vi "1_3oct_extrator_csv_to_csv.vi"() -> ()   [LabVIEW 2017]
doc: "Permite obtener un archivo CSV de etiquetado automático de secciones de señal. \nIngresa: un archivo CSV que contiene el sample inicial, final y la etiqueta correspondiente.\nUn archivo TDMS que contenga la información del registro de la señal.\nSe debe colocar la dirección del archivo de salida.\nEstablecer el número de samples que contendrá cada parte en que se dividirá la sección.\nAl momento el VI no contempla traslapamiento."
uses:
  <vilib>/Waveform/WDTOps.llb/WDT Get Waveform Subset DBL.vi
  <vilib>/addons/Sound and Vibration/svt_Octave_2014 standard/SVT Third-octave Analysis (1 Ch).vi
  <vilib>/addons/Sound and Vibration/svt_Level/SVT Sound Level (1 Ch).vi
  <vilib>/Utility/file.llb/Write Delimited Spreadsheet (string).vi
  <vilib>/addons/Sound and Vibration/svt_Octave/SoundVib_Octave_2014 standard.lvlib
  <vilib>/addons/Sound and Vibration/svt_Level/SoundVib_SoundLevel.lvlib
panel:
  out "F-format string":string[][](array[string])
  out "Array":dbl[][](array[numeric])
  out "Dynamic Data Type":dbl
  in  "Canal":string[](array[string])=["Sound Pressure_0"]
  out "Para el CSV, excepto fecha y hora":string[][](array[string])
  out "TIEMPOS":timestamp[](array[timestamp])
  out "Objetos por sección.":i32[][](array[numeric])
  out "Objetos":i32[](array[numeric])
  out "Secciones":i32[](array[numeric])
  out "Objetos totales":i32
  in  "frequency range":T1={"low band"=enum."20 Hz", "high band"=enum."20000 Hz"}
  out "TO CSV.":string[][](array[string])
  out "ETIQUETAS":string[](array[string])
  out "BANDAS":dbl[][](array[numeric])
  in  "ETIQUETADO":path=path "C:/Users/CRamos/Documents/MATLAB/etiquetador/csv_OUT/DATOS_caracte.csv"
  out "Objeto actual":i32
  out "Sección Actual":i32
  out "Samples \npor Objeto":waveform(dbl)
  in  "Largo de ventada temporal en N samples":dbl=4410.0
  out "Secciones":waveform(dbl)[](array[waveform])
  out "Multiplot \noctave graph":T2(graph)
  in  "ARCHIVO\nTDMS":path=path "C:/Users/CRamos/Documents/MATLAB/TDMS_files/two_sounds.tdms"
  in  "Archivo de\nreferencias (.csv)":path=path "C:/Users/CRamos/Documents/MATLAB/etiquetador/csv_IN/DATOS.csv"
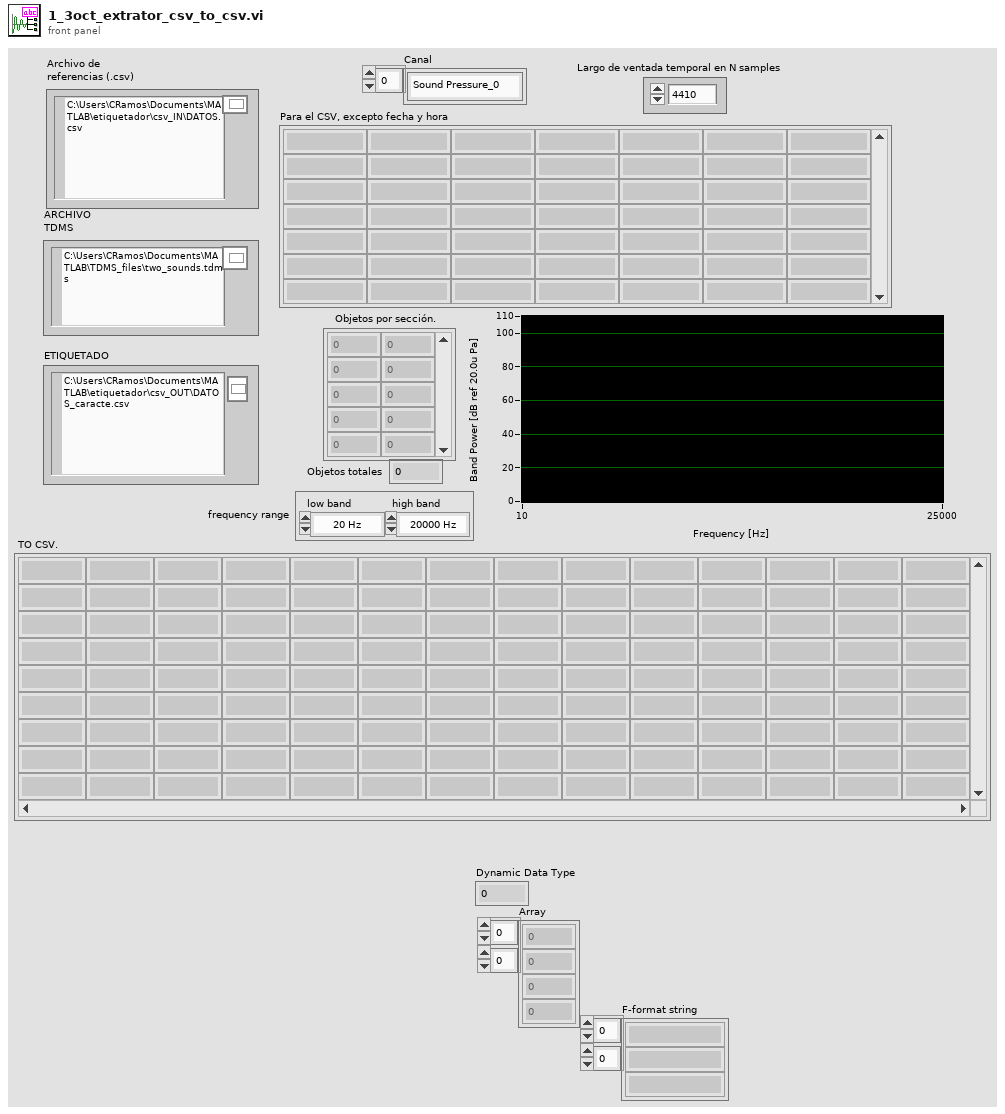
[diagram p1: front panel]
types:
  T1 = cluster{"low band":enum16{"20 Hz", "25 Hz", "31.5 Hz", "40 Hz", "50 Hz", "63 Hz", "80 Hz", "100 Hz", "125 Hz", "160 Hz", "200 Hz", "250 Hz", "315 Hz", "400 Hz", "500 Hz", "630 Hz", "800 Hz", "1000 Hz", "1250 Hz", "1600 Hz", "2000 Hz", "2500 Hz", "3150 Hz", "4000 Hz", "5000 Hz", "6300 Hz", "8000 Hz", "10000 Hz", "12500 Hz", "16000 Hz", "20000 Hz"}, "high band":enum16{"20 Hz", "25 Hz", "31.5 Hz", "40 Hz", "50 Hz", "63 Hz", "80 Hz", "100 Hz", "125 Hz", "160 Hz", "200 Hz", "250 Hz", "315 Hz", "400 Hz", "500 Hz", "630 Hz", "800 Hz", "1000 Hz", "1250 Hz", "1600 Hz", "2000 Hz", "2500 Hz", "3150 Hz", "4000 Hz", "5000 Hz", "6300 Hz", "8000 Hz", "10000 Hz", "12500 Hz", "16000 Hz", "20000 Hz"}}
  T2 = cluster{"nominal frequencies [Hz]":dbl[], "band power":dbl[]}
  T3 = enum16{"open", "open or create", "create or replace", "create", "open (read-only)"}
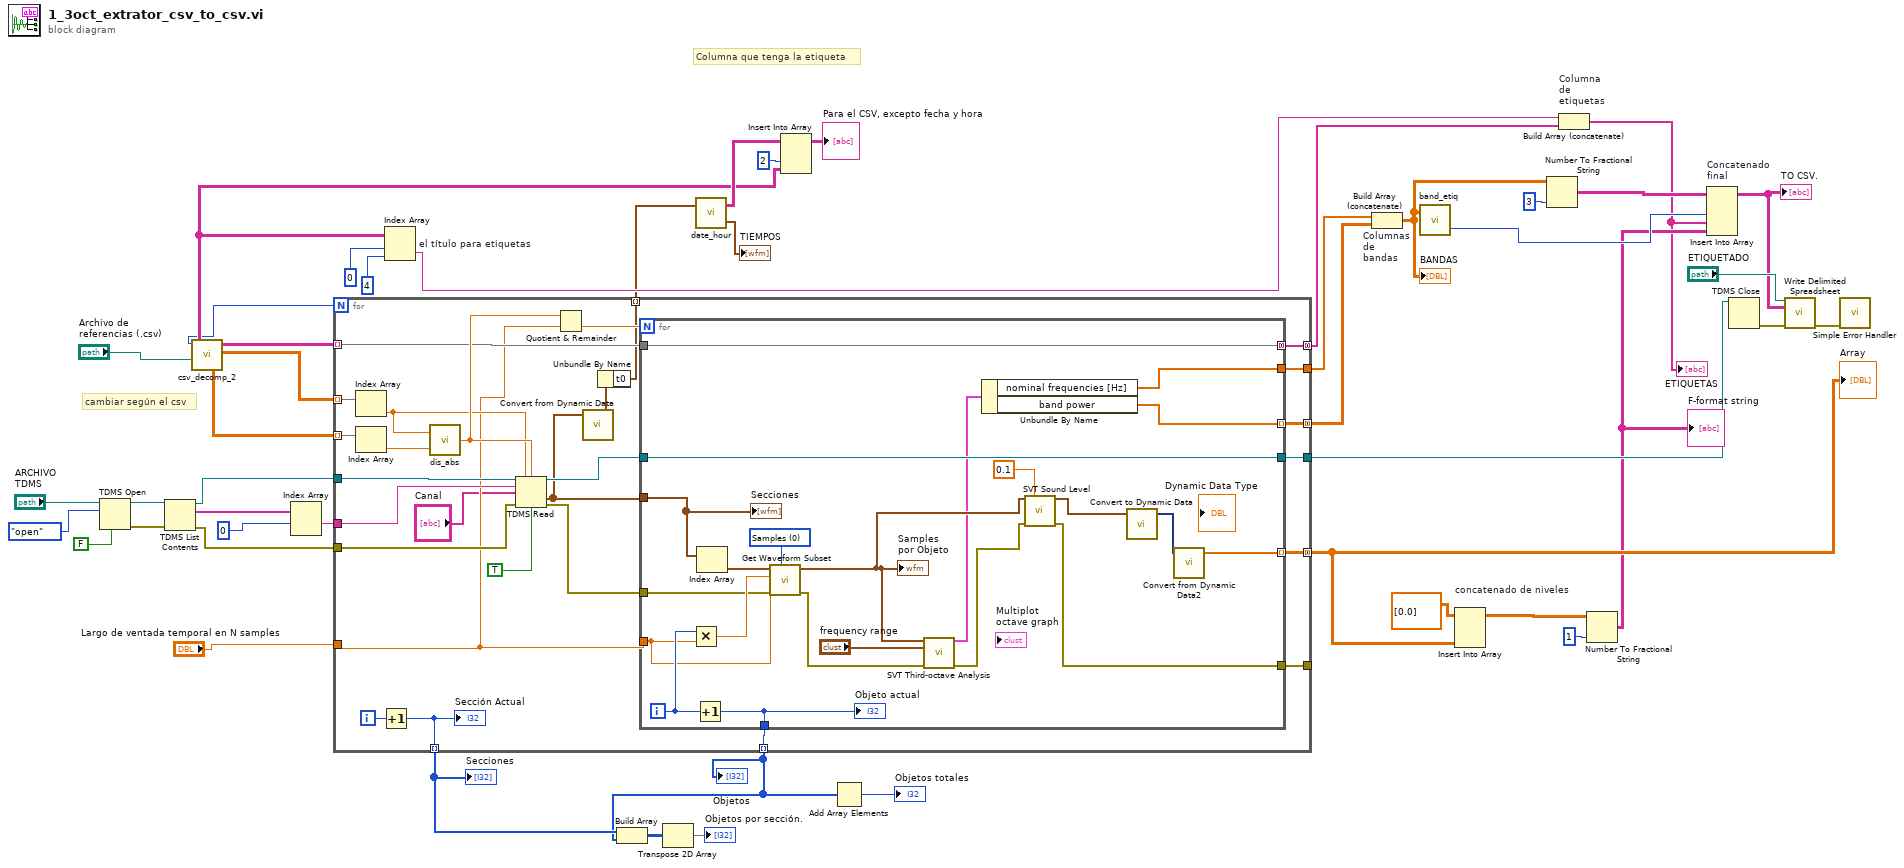
[diagram p0: block diagram]
diagram:
  # "cambiar según el csv"
  # "Columna que tenga la etiqueta"
  n1 = TDMS Open(6:FALSE ("disable buffering? (T)"), 10:T3."open" ("operation (0:open)"), 11:"ARCHIVO\nTDMS") -> (0:w45:errorcluster, 3:w16:refnum<k34>)  [unwired: 4 in]
  n2 = TDMS List Contents(4:w45, 7:w16) -> (0:w14:errorcluster, 2:w15:string[], 3:w44:refnum<k34>)  [unwired: 1 in, 1 out]
  n3 = call "csv_decomp_2.vi"("Archivo de referencias (.csv)"="Archivo de\nreferencias (.csv)") -> ("finales"=w9:dbl[][], "iniciales"=w8:dbl[][], "etiquetas"=w10:string[][], "# dimención"=w11:i32, "Lectura CSV"=w13:string[][])  [unwired: 2 in]
  n4 = Index Array(array=w15, index #1=0 ("index")) -> (element #1=w42:string)  [unwired: 1 in, 1 out]
  n5 = for {
    N: w11 -> [_]
    tunnel: w8 -> [w72] mode=indexing
    tunnel: w9 -> [w73] mode=indexing
    tunnel: w10 -> [w60] mode=indexing
    tunnel: w44 -> [w74]
    tunnel: w14 -> [w67]
    tunnel: w42 -> [w75]
    tunnel: [w65] -> w41
    tunnel: [w63] -> w40
    tunnel: [w62] -> w39 mode=concatenating
    tunnel: [w61] -> _
    tunnel: [w59] -> w35 mode=concatenating
    tunnel: [w58] -> w24 mode=indexing
    tunnel: "Largo de ventada temporal en N samples" -> [w55]
    tunnel: [w54] -> w25 mode=indexing
    tunnel: [w51] -> w21 mode=indexing
    tunnel: [w49] -> w6 mode=concatenating
    i -> [w64]
    n6 = Index Array(array=w72) -> (element=w57:dbl)  [unwired: 1 in]
    n7 = Index Array(array=w73) -> (element=w56:dbl)  [unwired: 1 in]
    n8 = Increment(x=w64) -> (x+1=w54:i32)
    "Sección Actual" <- w54
    n9 = call "dis_abs.vi"("Numeric in"=w56, "Numeric 3"=w57) -> ("distancia abs entre dos números"=w68:dbl)
    n10 = TDMS Read(0:w74, 1:w57, 2:w68, 5:w75, 7:"Canal", 11:w67, 13:TRUE ("return channels in file order? (F)")) -> (4:w71:refnum<k34>, 10:w53:waveform(dbl)[], 15:w66:errorcluster)  [unwired: 1 in, 3 out]
    n11 = Quotient & Remainder(x=w68, y=w55) -> (floor(x/y)=w69:dbl)  [unwired: 1 out]
    n12 = call "Convert from Dynamic Data"("Dynamic Data Type"=w53) -> ("Waveform"=w52:waveform(dbl))  [unwired: 3 in]
    n13 = Unbundle By Name(w52) -> ("t0"=w51:timestamp)
    n14 = for {
      N: w69 -> [_]
      tunnel: w71 -> [w92]
      tunnel: w53 -> [w84]
      tunnel: w66 -> [w93]
      tunnel: [w81] -> w61
      tunnel: [w92] -> w65
      tunnel: [w91] -> w63
      tunnel: [w90] -> w62 mode=indexing
      tunnel: w60 -> [w89]
      tunnel: [w89] -> w59 mode=concatenating
      tunnel: [w87] -> w58
      tunnel: w55 -> [w85]
      tunnel: [w76] -> w49 mode=indexing
      i -> [w86]
      w95 = u16 0 items=["Samples", "Relative Time"] ("start/duration format")
      n15 = Multiply(x=w86, y=w85) -> (x*y=w94:dbl)
      n16 = Increment(x=w86) -> (x+1=w87:i32)
      "Objeto actual" <- w87
      n17 = Index Array(array=w84) -> (element=w96:waveform(dbl))  [unwired: 1 in]
      n18 = call-poly <vilib>:"Get Waveform Subset.vi"("start/duration format"=w95, "error in (no error)"=w93, "duration"=w85, "start samples/time"=w94, "waveform in"=w96) -> ("error out"=w97:errorcluster, "waveform out"=w83:waveform(dbl))  [unwired: 1 in, 2 out]
      "Samples \npor Objeto" <- w83
      n19 = call-poly <vilib>:"SVT Third-octave Analysis.vi"("scaled signal [EU]"=w83, "frequency range"="frequency range", "error in (no error)"=w97) -> ("octave spectrum"=w79:T2, "error out"=w82:errorcluster)  [unwired: 7 in, 4 out]
      n20 = Unbundle By Name(w79) -> ("nominal frequencies [Hz]"=w91:dbl[], "band power"=w90:dbl[])
      n21 = call-poly <vilib>:"SVT Sound Level.vi"("scaled signal [EU]"=w83, "integration time [s]"=0.1, "error in (no error)"=w82) -> ("Leq sound level [dB EU]"=w78:waveform(dbl), "error out"=w81:errorcluster)  [unwired: 7 in, 4 out]
      n22 = call "Convert to Dynamic Data"("Array"=w78) -> ("Dynamic Data Type"=w77:dynamicdata)  [unwired: 3 in]
      n23 = call "Convert from Dynamic Data2"("Dynamic Data Type"=w77) -> ("Array"=w76:dbl[])  [unwired: 3 in]
      "Secciones" <- w84
    }
  }
  "Secciones" <- w25
  "Objetos" <- w24
  "Array" <- w6
  n24 = Index Array "el título para etiquetas"(array=w13, index (row)=0 ("disabled index (row)"), index (col)=4 ("disabled index (col)")) -> (element=w32:string)
  n25 = Build Array(w25, w24) -> (w23:i32[][])
  n26 = Transpose 2D Array(2D array=w23) -> (transposed array=→"Objetos por sección.":i32[][])
  n27 = call "date_hour.vi"("Array"=w21) -> ("date/hour"=→"TIEMPOS":timestamp[], "appended array"=w19:string[][])  [unwired: 1 in]
  n28 = Insert Into Array(array=w19, index (col)=2 ("disabled index (col)"), new element=w13) -> (→"Para el CSV, excepto fecha y hora":string[][])  [unwired: 1 in]
  n29 = Add Array Elements(numeric array=w24) -> (sum=→"Objetos totales":i32)
  n30 = Build Array (concatenate) "Columnas \nde\nbandas"(w40, w39) -> (w29:dbl[][])
  "BANDAS" <- w29
  n31 = call "band_etiq.vi"("Array de entrada"=w29) -> ("Numeric"=w28:i32)  [unwired: 1 in, 1 out]
  n32 = Insert Into Array "concatenado de niveles"(array=dbl[][] [[0.0]], new element=w6) -> (w5:dbl[][])  [unwired: 2 in]
  n33 = Number To Fractional String(number=w29, precision (6)=i16 3) -> (F-format string=w30:string[][])  [unwired: 2 in]
  n34 = Build Array (concatenate) "Columna \nde \netiquetas"(w32, w35) -> (w1:string[])
  "ETIQUETAS" <- w1
  n35 = Number To Fractional String(number=w5, precision (6)=i16 1) -> (F-format string=w3:string[][])  [unwired: 2 in]
  "F-format string" <- w3
  n36 = Insert Into Array "Concatenado \nfinal"(array=w30, index (col)=w28, new element #1=w1, new element #2=w3) -> (w2:string[][])  [unwired: 1 in]
  "TO CSV." <- w2
  n37 = TDMS Close(11:w41) -> (0:w37:errorcluster)  [unwired: 1 in, 1 out]
  n38 = call-poly <vilib>:"Write Delimited Spreadsheet.vi"("file path (dialog if empty)"="ETIQUETADO", "2D data"=w2, "error in (no error)"=w37) -> ("error out"=w36:errorcluster)  [unwired: 11 in, 1 out]
  n39 = call <vilib>:"Simple Error Handler.vi"("error in (no error)"=w36) -> ()  [unwired: 4 in, 5 out]
